vi "Gyro Read.vi"(8 "error in (no error)":errorcluster, 11 "I2CDevRef In":T2={"DevStatus"={"status"=FALSE, "code"=0, "source"=""}, "Device Address"=0, "Handle"=0, "I2C Bus"=enum."Invalid"} {"Device Address" format="%.0x"}) -> (0 "error out":errorcluster, 2 "Angular Rate":dbl, 3 "Angle":dbl)   [LabVIEW 2015]
uses:
  <vilib>/Rock Robotics/WPI/I2C/WPI_I2CDevRef.ctl
  <vilib>/Rock Robotics/SystemInterfaces/i2clib/i2c_bus.ctl
  DPS Mode.ctl
  Gyro Globals.vi
panel:
  out "Current Field Angle":dbl(graph)
  out "DPS Mode":T1
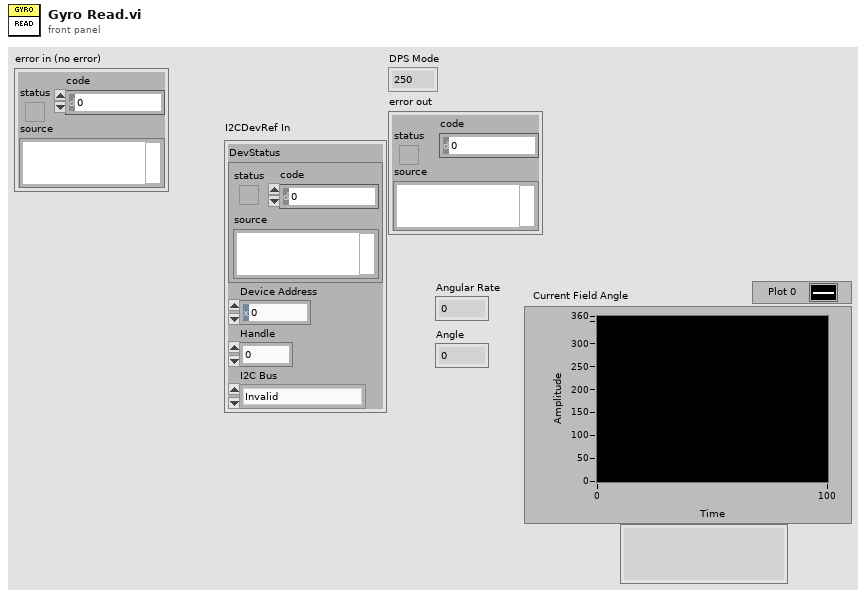
[diagram p1: front panel]
types:
  T1 = typedef "DPS Mode.ctl" = enum16{"250", "500", "2000"}
  T2 = typedef "WPI_I2CDevRef.ctl" = cluster{"DevStatus":errorcluster, "Device Address":u8, "Handle":i32, "I2C Bus":T3}
  T3 = typedef "i2c_bus.ctl" = enum16{"I2C On-Board", "I2C MXP", "Invalid"}
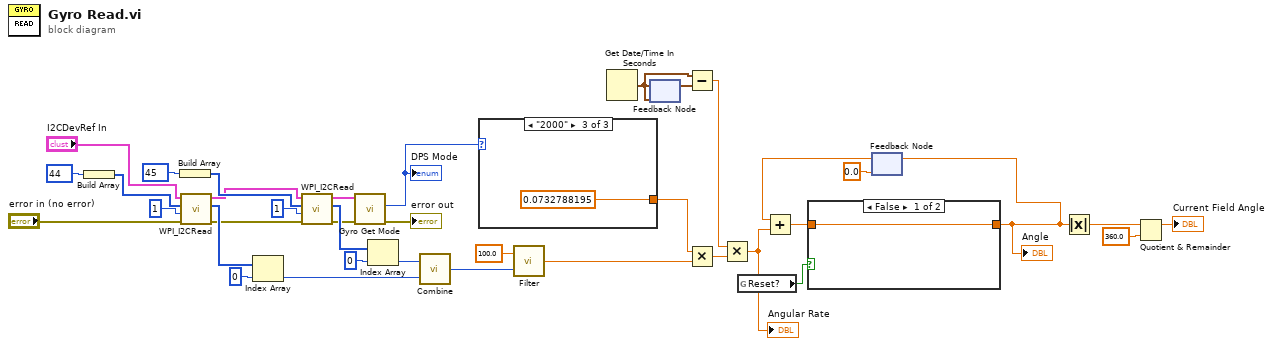
[diagram p0: block diagram]
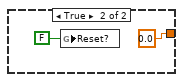
[diagram p2: hidden frame]
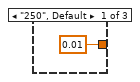
[diagram p3: hidden frame]
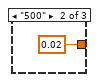
[diagram p4: hidden frame]
diagram:
  n1 = Build Array(u8 44 ("Data To Send")) -> (w37:u8[])
  n2 = Build Array(u8 45 ("Data To Send")) -> (w33:u8[])
  n3 = call <vilib>:"WPI_I2CRead.vi"("error in (no error)"="error in (no error)", "I2CBytesToRead"=u8 1, "I2CRegister"=w37, "I2CDevRef"="I2CDevRef In") -> ("error out"=w9:errorcluster, "Data Out"=w30:u8[], "I2CDevRef"=w31:T2)  [unwired: 5 in]
  n4 = Index Array(array=w30, index=0) -> (element=w25:u8)
  n5 = call <vilib>:"WPI_I2CRead.vi"("error in (no error)"=w9, "I2CBytesToRead"=u8 1, "I2CRegister"=w33, "I2CDevRef"=w31) -> ("error out"=w8:errorcluster, "Data Out"=w27:u8[], "I2CDevRef"=w16:T2)  [unwired: 5 in]
  n6 = call "Gyro Get Mode.vi"("error in (no error)"=w8, "I2CDevRef"=w16) -> ("error out"=→"error out":errorcluster, "DPS Mode"=w15:T1)  [unwired: 7 in, 1 out]
  "DPS Mode" <- w15
  n7 = Index Array(array=w27, index=0) -> (element=w26:u8)
  n8 = call "Combine.vi"("L"=w25, "H"=w26) -> ("Out"=w24:i16)
  n9 = case shown="\"2000\"" w15 {
    tunnel: [0.01 ("Gyro Gain") 0.02 ("Gyro Gain") 0.0732788195 ("Gyro Gain")] -> w14
    frame "250", Default {
    }
    frame "500" {
    }
    frame "2000" {
    }
  }
  n10 = call "Filter.vi"("In"=w24, "Window"=100.0) -> ("Out"=w21:dbl)
  n11 = Get Date/Time In Seconds() -> (seconds since 1Jan1904=w1:timestamp)
  n12 = feedback-in #1(w1) -> ()
  n13 = feedback #1(w1) -> (w11:timestamp)
  n14 = Subtract(x=w1, y=w11) -> (x-y=w10:dbl)
  n15 = Multiply(x=w14, y=w21) -> (x*y=w22:dbl)
  n16 = Multiply(x=w10, y=w22) -> (x*y=w19:dbl)
  "Angular Rate" <- w19
  n17 = global read "Gyro Globals.vi" "Reset?"() -> (w13:bool)
  n18 = feedback #2(0.0) -> (w18:dbl)
  n19 = Add(x=w18, y=w19) -> (x+y=w12:dbl)
  n20 = case shown="False" w13 {
    tunnel: w12 -> [w41 _]
    tunnel: [w41 0.0] -> w4
    frame False {
    }
    frame True {
      n21 = global write "Gyro Globals.vi" "Reset?"(FALSE ("Reset?")) -> ()
    }
  }
  "Angle" <- w4
  n22 = feedback-in #2(w4) -> ()
  n23 = Absolute Value(x=w4) -> (abs(x)=w5:dbl)
  n24 = Quotient & Remainder(x=w5, y=360.0) -> (x-y*floor(x/y)=→"Current Field Angle":dbl)  [unwired: 1 out]
